vi "Incomplete Analysis Type Selection.vi"(8 "Error In":errorcluster) -> (0 "Error Out":errorcluster, 3 "Yes or No":string)   [LabVIEW 2020]
panel:
  in  "NO":bool
  in  "YES":bool
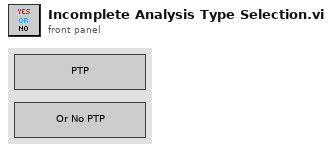
[diagram p1: front panel]
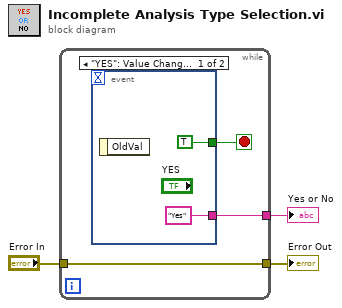
[diagram p0: block diagram]
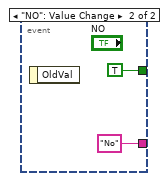
[diagram p2: hidden frame]
diagram:
  n1 = while {
    tunnel: [w5] -> w3
    tunnel: "Error In" -> [w4]
    tunnel: [w4] -> w1
    stop <- w6 stop-if-true
    n2 = event shown="[0] \"YES\": Value Change" {
      selector: _ -> [_ _]
      dyn-events: _ -> [_ _]
      timeout: _ -> [_ _]
      tunnel: [TRUE TRUE] -> w6
      tunnel: ["Yes" "No"] -> w5
      event "YES": Value Change {
        n3 = event-data() -> ()  [unwired: 1 in, 1 out]
      }
      event "NO": Value Change {
        n4 = event-data() -> ()  [unwired: 1 in, 1 out]
      }
    }
  }
  "Yes or No" <- w3
  "Error Out" <- w1
